vi "Flip Tile Horizontal.vi"(8 "error in (no error)":errorcluster, 11 "Tile in":refnum<class "Tile.lvclass">) -> (0 "error out":errorcluster, 3 "Tile out":refnum<class "Tile.lvclass">)   [LabVIEW 2020, in "Tile.lvclass"]
uses:
  Tile.lvclass
  Tile.lvclass/Tile.ctl
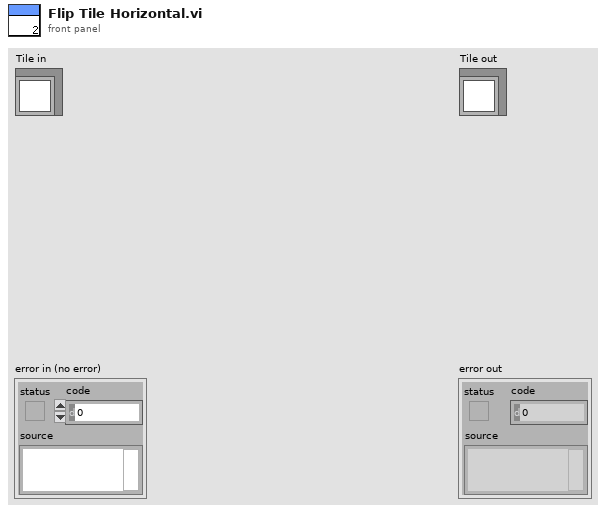
[diagram p1: front panel]
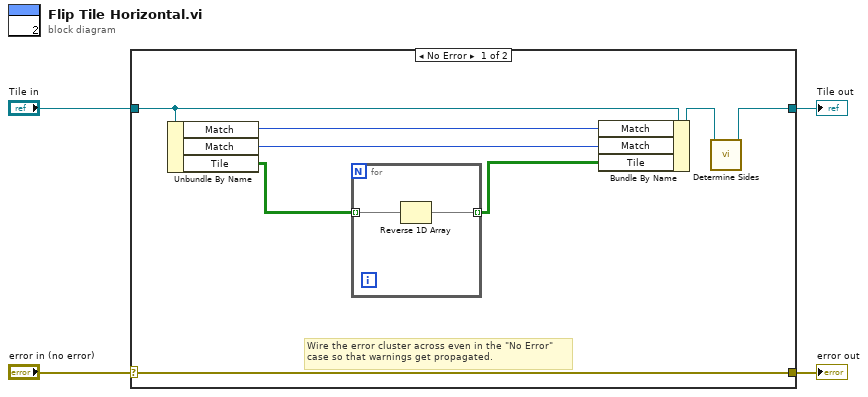
[diagram p0: block diagram]
diagram:
  n1 = case shown="No Error" "error in (no error)" {
    selector: "error in (no error)" -> [w12 w16]
    tunnel: [w12 w16] -> w3
    tunnel: [w8 w15] -> w1
    tunnel: "Tile in" -> [w10 w15]
    frame No Error {
      # "Wire the error cluster across even in the \"No Error\"\ncase so that warnings get propagated."
      n2 = Unbundle By Name(w10) -> ("Match"=w6:u64, "Match"=w7:u64, "Tile"=w11:bool[][])
      n3 = for {
        tunnel: w11 -> [w14] mode=indexing
        tunnel: [w13] -> w5 mode=indexing
        n4 = Reverse 1D Array(array=w14) -> (reversed array=w13:bool[])
      }
      n5 = Bundle By Name(cluster=w10, "Match"=w6, "Match"=w7, "Tile"=w5) -> (w9:refnum<class "Tile.lvclass">)
      n6 = call "Determine Sides.vi"("Tile in"=w9) -> ("Tile out"=w8:refnum<class "Tile.lvclass">)  [unwired: 9 in, 1 out]
    }
    frame Error {
    }
  }
  "error out" <- w3
  "Tile out" <- w1
